vi "GT Get Home Status.vi"(8 "error in (no error)":errorcluster caption="错误输入（无错误）", 10 "axis":i16, 11 "cardNum":i16) -> (0 "error out":errorcluster caption="错误输出", 1 "pHomeStatus out":T1, 3 "cardNum":i16)   [LabVIEW 2020, in "gts.lvlib"]
doc: "GT_API GT_GetHomeStatus(short cardNum,short axis,THomeStatus *pHomeStatus);"
uses:
  gts.lvlib
  Controls/HomeStatus.ctl
  dll/32bit/multi_card/gts.dll
  Controls/Controls.lvlib
panel:
  # "{\nshort run; // 是正在进行回原点，0—已停止运动，1-正在回\n原点\nshort stage; // 回原点运动的阶段\nshort error; // 回原点过程的发生的错误\nshort pad1; // 保留（无具体含义）\nlong capturePos; // 捕获到Home或Index时刻的编码器位置\nlong targetPos; // 需要运动到的目标位置（原点位置或者原点\n位置+偏移量），在搜索Limit时或者搜索Home\n或Index时，设置的搜索距离为0，那么该值显示\n为805306368\n} THomeStatus;"
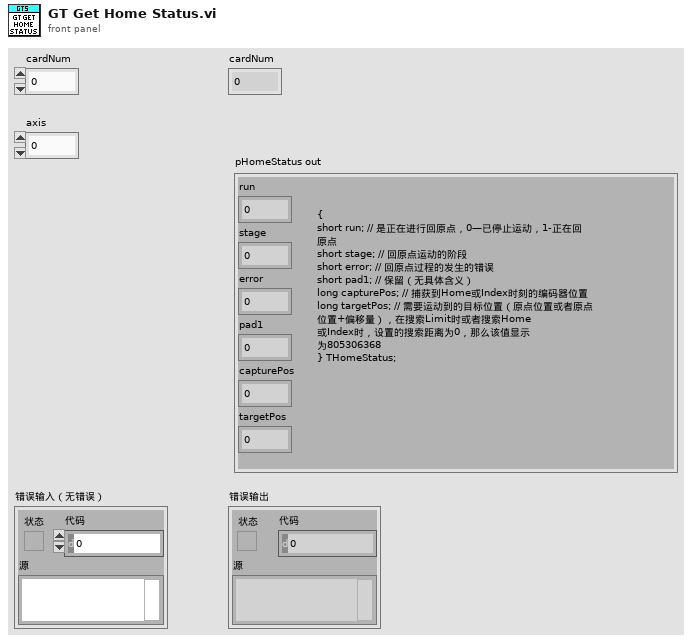
[diagram p1: front panel]
types:
  T1 = typedef "Controls.lvlib/HomeStatus.ctl" = cluster{"run":i16, "stage":i16, "error":i16, "pad1":i16, "capturePos":i32, "targetPos":i32}
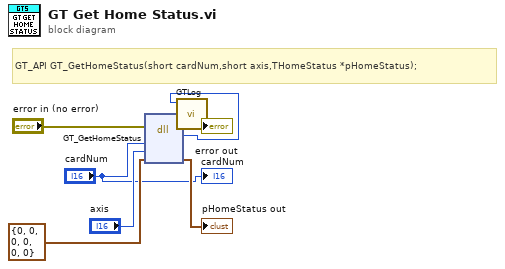
[diagram p0: block diagram]
diagram:
  # "GT_API GT_GetHomeStatus(short cardNum,short axis,THomeStatus *pHomeStatus);"
  n1 = dll-call lib="D:/Git/GoogolCard/dll/32bit/multi_card/gts.dll" fn="GT_GetHomeStatus"(error in="error in (no error)", "cardNum"="cardNum", "axis"="axis", "pHomeStatus"=T1 {"run"=0, "stage"=0, "error"=0, "pad1"=0, "capturePos"=0, "targetPos"=0}) -> (error out=w4:errorcluster, w2:i16, "pHomeStatus"=→"pHomeStatus out":T1)  [unwired: 4 in, 1 out]
  n2 = call "GTLog.vi"("error in (no error)"=w4, "Numeric"=w2) -> ("error out"=→"error out":errorcluster)  [unwired: 9 in]
  "cardNum" <- "cardNum"
